vi "Lift_Function.vi"(6 "Low Range":T14, 7 "High Range":T15, 9 "Input Cluster":T16={"Level 5"=TRUE, "Level 4"=TRUE, "Level 3"=TRUE, "Level 2"=TRUE, "Level 1"=FALSE}) -> (3 "Output Cluster":T16)   [LabVIEW 2014]
uses:
  <vilib>/Rock Robotics/WPI/PWM/WPI_PWMTransform_ConPane.ctl
  <vilib>/Rock Robotics/WPI/CAN/Jaguar/SubVIs/WPI_CANJaguar_ControlMode.ctl
  <vilib>/Rock Robotics/WPI/CAN/TalonSRX/WPI_CANTalonSRX_APIControlMode.ctl
  <vilib>/Rock Robotics/SystemInterfaces/Typedef/FPGA_TypedefDigitalModule.ctl
  <vilib>/Rock Robotics/SystemInterfaces/DIO/FPGA_DIOPWMChannel.ctl
  <vilib>/Rock Robotics/WPI/PWM/WPI_PWMDeadband.ctl
  <vilib>/Rock Robotics/WPI/MotorControl/WPI_MotorControlType.ctl
  <vilib>/Rock Robotics/WPI/MotorControl/WPI_MotorControlDeviceRef.ctl
  <vilib>/Rock Robotics/SystemInterfaces/Encoder/FPGA_EncoderIdx.ctl
  <vilib>/Rock Robotics/WPI/Encoder/WPI_EncoderType.ctl
  <vilib>/Rock Robotics/SystemInterfaces/Counter/FPGA_CounterCtrSystemIndex.ctl
  <vilib>/Rock Robotics/WPI/Encoder/WPI_EncoderDevRef.ctl
panel:
  in  "EncoderDevRef":T1={"DevStatus"={"status"=FALSE, "code"=0, "source"=""}, "EncoderIndex"=enum."Invalid", "CounterIndex"=enum."Invalid", "DistancePerCount"=1.0, "Decoding Type"=enum."4x"}
  in  "MotorControlDevRef":T5={"DeviceStatus"={"status"=FALSE, "code"=0, "source"=""}, "Type"=enum."PWM", "PWM"={"Controller"=enum."Controller 1", "PWM Channel"=enum."Invalid", "DeadBand"={"Name"="", "maxPositivePwm"=0, "minPositivePwm"=0, "centerPwm"=0, "maxNegativePwm"=0, "minNegativePwm"=0, "angularRange"=0}}, "CAN"={"Device Number"=0, "Control Mode"=enum."Percent VBus", "Semaphore"=refnum, "Max Vout"=12.0, "TalonSRX Control Mode"=enum."Percent VBus"}, "Invert"=FALSE, "TransformRef"=refnum, "InvTransformRef"=refnum}
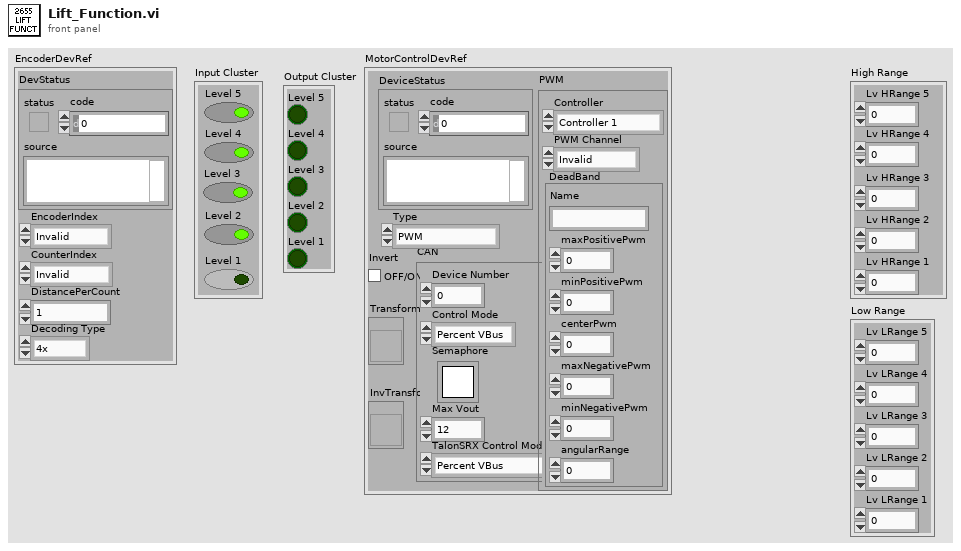
[diagram p1: front panel]
types:
  T1 = typedef "WPI_EncoderDevRef.ctl" = cluster{"DevStatus":errorcluster, "EncoderIndex":T2, "CounterIndex":T3, "DistancePerCount":dbl, "Decoding Type":T4}
  T2 = typedef "FPGA_EncoderIdx.ctl" = enum8{"Enc 0", "Enc 1", "Enc 2", "Enc 3", "Enc 4", "Enc 5", "Enc 6", "Enc 7", "Invalid"}
  T3 = typedef "FPGA_CounterCtrSystemIndex.ctl" = enum8{"Ctr 0", "Ctr 1", "Ctr 2", "Ctr 3", "Ctr 4", "Ctr 5", "Ctr 6", "Ctr 7", "Invalid"}
  T4 = typedef "WPI_EncoderType.ctl" = enum16{"1x", "2x", "4x"}
  T5 = typedef "WPI_MotorControlDeviceRef.ctl" = cluster{"DeviceStatus":errorcluster, "Type":T6, "PWM":cluster{"Controller":T7, "PWM Channel":T8, "DeadBand":T9}, "CAN":cluster{"Device Number":u8, "Control Mode":T10, "Semaphore":T11, "Max Vout":dbl, "TalonSRX Control Mode":T12}, "Invert":bool, "TransformRef":T13, "InvTransformRef":T13}
  T6 = typedef "WPI_MotorControlType.ctl" = enum16{"PWM", "CAN", "CANTalonSRX"}
  T7 = typedef "FPGA_TypedefDigitalModule.ctl" = enum16{"Controller 1"}
  T8 = typedef "FPGA_DIOPWMChannel.ctl" = enum8{"PWM 0", "PWM 1", "PWM 2", "PWM 3", "PWM 4", "PWM 5", "PWM 6", "PWM 7", "PWM 8", "PWM 9", "PWM MXP 0", "PWM MXP 1", "PWM MXP 2", "PWM MXP 3", "PWM MXP 4", "PWM MXP 5", "PWM MXP 6", "PWM MXP 7", "PWM MXP 8", "PWM MXP 9", "Invalid"}
  T9 = typedef "WPI_PWMDeadband.ctl" = cluster{"Name":string, "maxPositivePwm":i32, "minPositivePwm":i32, "centerPwm":i32, "maxNegativePwm":i32, "minNegativePwm":i32, "angularRange":u16}
  T10 = typedef "WPI_CANJaguar_ControlMode.ctl" = enum8{"Percent VBus", "Current", "Speed", "Position", "Voltage"}
  T11 = typedef "Semaphore RefNum" = refnum<k1>
  T12 = typedef "WPI_CANTalonSRX_APIControlMode.ctl" = enum8{"Percent VBus", "Speed", "Position", "Slave", "Unchanged / Invalid"}
  T13 = typedef "WPI_PWMTransform_ConPane.ctl" = refnum<vi>
  T14 = cluster{"Lv LRange 1":dbl, "Lv LRange 2":dbl, "Lv LRange 3":dbl, "Lv LRange 4":dbl, "Lv LRange 5":dbl}
  T15 = cluster{"Lv HRange 5":dbl, "Lv HRange 4":dbl, "Lv HRange 3":dbl, "Lv HRange 2":dbl, "Lv HRange 1":dbl}
  T16 = cluster{"Level 5":bool, "Level 4":bool, "Level 3":bool, "Level 2":bool, "Level 1":bool}
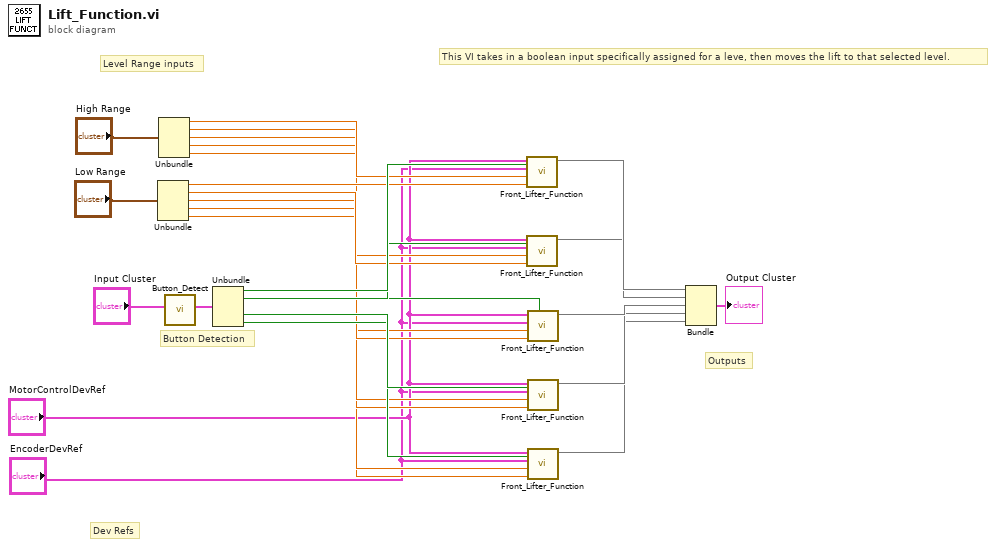
[diagram p0: block diagram]
diagram:
  # "This VI takes in a boolean input specifically assigned for a leve, then moves the lift to that selected level."
  # "Button Detection"
  # "Outputs"
  # "Dev Refs"
  # "Level Range inputs"
  n1 = Unbundle("Low Range") -> ("Lv LRange 1"=w11:dbl, "Lv LRange 2"=w10:dbl, "Lv LRange 3"=w8:dbl, "Lv LRange 4"=w6:dbl, "Lv LRange 5"=w4:dbl)
  n2 = Unbundle("High Range") -> ("Lv HRange 5"=w12:dbl, "Lv HRange 4"=w9:dbl, "Lv HRange 3"=w3:dbl, "Lv HRange 2"=w7:dbl, "Lv HRange 1"=w5:dbl)
  n3 = call "Button_Detect.vi"("Input Cluster"="Input Cluster") -> ("Output Cluster"=w21:T16)  [unwired: 10 in]
  n4 = Unbundle(w21) -> ("Level 5"=w20:bool, "Level 4"=w19:bool, "Level 3"=w18:bool, "Level 2"=w17:bool, "Level 1"=w16:bool)
  n5 = call "Front_Lifter_Function.vi"(7:w20, 8:w11, 9:w12, "Go to Level?"="EncoderDevRef", 11:"MotorControlDevRef") -> (3:w27)  [unwired: 4 in, 2 out]
  n6 = call "Front_Lifter_Function.vi"(7:w19, 8:w10, 9:w9, "Go to Level?"="EncoderDevRef", 11:"MotorControlDevRef") -> (3:w26)  [unwired: 4 in, 2 out]
  n7 = call "Front_Lifter_Function.vi"(7:w18, 8:w8, 9:w3, "Go to Level?"="EncoderDevRef", 11:"MotorControlDevRef") -> (3:w25)  [unwired: 4 in, 2 out]
  n8 = call "Front_Lifter_Function.vi"(7:w17, 8:w6, 9:w7, "Go to Level?"="EncoderDevRef", 11:"MotorControlDevRef") -> (3:w24)  [unwired: 4 in, 2 out]
  n9 = call "Front_Lifter_Function.vi"(7:w16, 8:w4, 9:w5, "Go to Level?"="EncoderDevRef", 11:"MotorControlDevRef") -> (3:w23)  [unwired: 4 in, 2 out]
  n10 = Bundle(w27, w26, w25, w24, w23) -> (→"Output Cluster":cluster{void, void, void, void, void})  [unwired: 1 in]
